vi "Local Configuration.LAS1BA.Local Base Address.Set.vi"(8 "error in (no error)":errorcluster, 10 "Local Base Address":u32 format="%.0x", 11 "GE 5565PIORC":refnum<class "GE 5565PIORC.lvclass">) -> (0 "error out":errorcluster, 3 "GE 5565PIORC out":refnum<class "GE 5565PIORC.lvclass">)   [LabVIEW 2016, in "GE 5565PIORC.lvclass"]
uses:
  GE 5565PIORC.lvclass
  <vilib>/Instr/_visa.llb/VISA Register Access Address Space.ctl
  Controls/Registers.Local Configuration.ctl
  GE 5565PIORC.lvclass/GE 5565PIORC.ctl
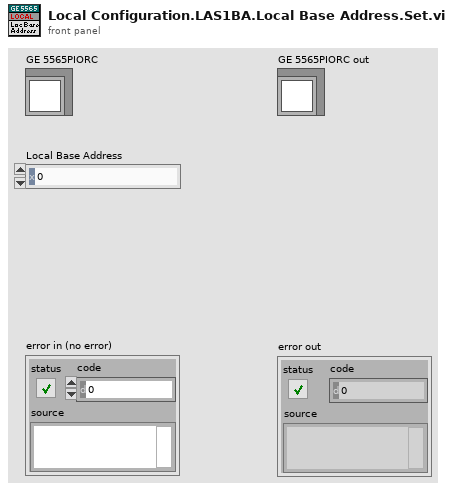
[diagram p1: front panel]
types:
  T1 = typedef "GE 5565PIORC.lvclass/Registers.Local Configuration.ctl" = enum16{"DMA Arbitration", "Interrupt Control and Status", "DMA Mode", "DMA PCI Address", "DMA Local Address", "DMA Transfer Size", "DMA Descriptor Pointer", "DMA Command/Status", "DMA PCI DAC Upper Address", "PCI PIO Address Range", "PCI PIO Base Address (Remap)"}
  T2 = typedef "VISA Register Access Address Space.ctl" = u16
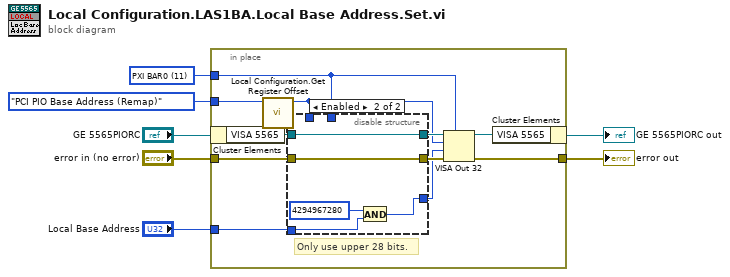
[diagram p0: block diagram]
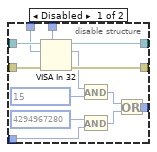
[diagram p2: hidden frame]
diagram:
  w2 = T2 11 items=["VXI/VME A16"=1, "VXI/VME A24"=2, "VXI/VME A32"=3, "VXI/VME A64"=4, "PXI Memory Allocations"=9, "PXI Configuration"=10, "PXI BAR0"=11, "PXI BAR1"=12, "PXI BAR2"=13, "PXI BAR3"=14, "PXI BAR4"=15, "PXI BAR5"=16] ("Address Space")
  n1 = in-place {
    in-place-border: "error in (no error)" -> [w17]
    in-place-border: [w13] -> w5
    in-place-border: Registers.Local_Configuration."PCI PIO Base Address (Remap)" ("Local Configration Register Offset") -> [w11]
    in-place-border: w2 -> [w10]
    in-place-border: "Local Base Address" -> [w8]
    # "Only use upper 28 bits."
    n2 = in-place-cluster #1("GE 5565PIORC") -> ("VISA 5565"=w18:refnum<visa-resource-name>)
    n3 = call "Local Configuration.Get Register Offset.vi"("Local Configuration Register"=w11) -> ("Offset"=w12:u32)  [unwired: 10 in]
    n4 = disable-structure shown="Enabled" {
      disable-tunnel: w18 -> [w31 w34]
      disable-tunnel: w17 -> [w30 w33]
      disable-tunnel: [w29 w34] -> w16
      disable-tunnel: [w28 w33] -> w15
      disable-tunnel: w12 -> [w27 _]
      disable-tunnel: w10 -> [w26 _]
      disable-tunnel: [w22 w32] -> w9
      disable-tunnel: w8 -> [w19 w35]
      frame Disabled {
        n5 = VISA In 32(7:w26, 8:w30, 10:w27, 11:w31) -> (0:w28:errorcluster, 2:w25:u32, 3:w29:refnum<visa-resource-name>)
        n6 = And(x=w25, y=u32 15 ("value")) -> (x .and. y?=w23:u32)
        n7 = And(x=u32 4294967280 ("value"), y=w19) -> (x .and. y?=w21:u32)
        n8 = Or(x=w23, y=w21) -> (x .or. y?=w22:u32)
      }
      frame Enabled {
        n9 = And(x=u32 4294967280 ("value"), y=w35) -> (x .and. y?=w32:u32)
      }
    }
    n10 = VISA Out 32(7:w10, 8:w15, 9:w9, 10:w12, 11:w16) -> (0:w13:errorcluster, 3:w14:refnum<visa-resource-name>)
    n11 = in-place-cluster #1("VISA 5565"=w14) -> (→"GE 5565PIORC out":refnum<class "GE 5565PIORC.lvclass">)
  }
  "error out" <- w5
